vi "XLP80_EA_Close Devices.vi"(8 "err in":errorcluster, 10 "Device Informations":T1, 11 "Simu EAs":T2) -> (0 "Error EAs":T3)   [LabVIEW 2021]
uses:
  XLP80_EA_TDefsCluster_EA Setpoint.ctl
  XLP80_EA_TDefsCluster_EA Setpoint_Reku.ctl
  XLP80_EA_Globals.vi
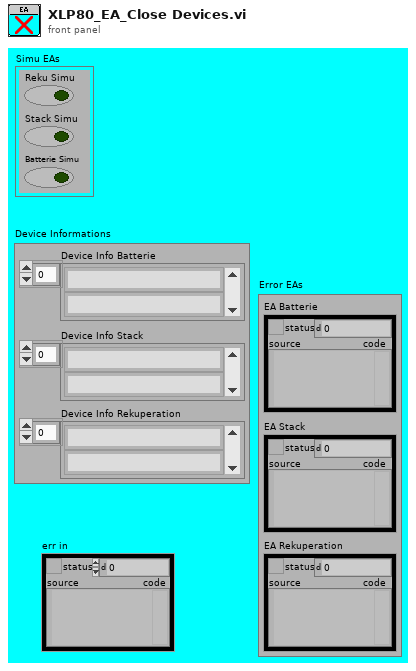
[diagram p1: front panel]
types:
  T1 = cluster{"Device Info Batterie":string[], "Device Info Stack":string[], "Device Info Rekuperation":string[]}
  T2 = cluster{"Reku Simu":bool, "Stack Simu":bool, "Batterie Simu":bool}
  T3 = cluster{"EA Batterie":errorcluster, "EA Stack":errorcluster, "EA Rekuperation":errorcluster}
  T4 = typedef "XLP80_EA_TDefsCluster_EA Setpoint_Reku.ctl" = cluster{"Load":bool, "Set Current":sgl, "Set Voltage":sgl, "Set Power":sgl}
  T5 = typedef "XLP80_EA_TDefsCluster_EA Setpoint.ctl" = cluster{"Load":bool, "Set Current":sgl, "Set Voltage":sgl}
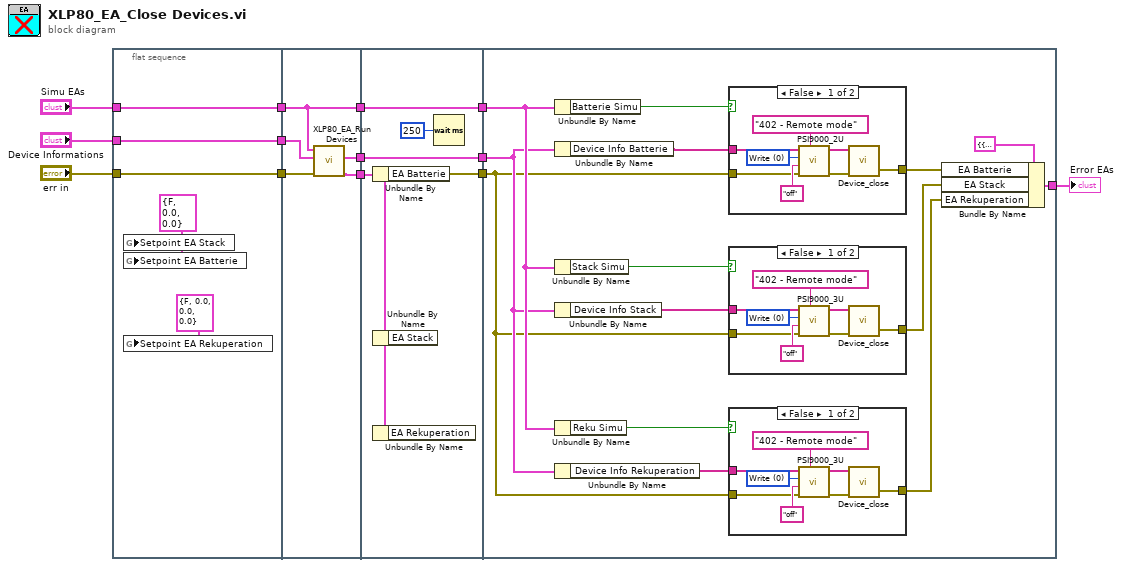
[diagram p0: block diagram]
diagram:
  n1 = flat-sequence {
    tunnel: "err in" -> [w16]
    tunnel: "Device Informations" -> [w17]
    tunnel: "Simu EAs" -> [w18]
    tunnel: [w18] -> w3
    tunnel: [w17] -> w2
    tunnel: [w16] -> w1
    tunnel: [w21] -> w6
    tunnel: [w20] -> w5
    tunnel: [w19] -> w4
    tunnel: w3 -> [w21]
    tunnel: w2 -> [w22]
    tunnel: w1 -> [w23]
    tunnel: [w28] -> w9
    tunnel: [w27] -> w8
    tunnel: [w26] -> w7
    tunnel: w6 -> [w28]
    tunnel: w5 -> [w27]
    tunnel: w4 -> [w25]
    tunnel: [w41] -> w13
    tunnel: w9 -> [w31]
    tunnel: w8 -> [w30]
    tunnel: w7 -> [w29]
    frame #0 {
      w15 = T5 {"Load"=FALSE, "Set Current"=0.0, "Set Voltage"=0.0} ("Setpoint EA Stack")
      n2 = global write "XLP80_EA_Globals.vi" "Setpoint EA Stack"(w15) -> ()
      n3 = global write "XLP80_EA_Globals.vi" "Setpoint EA Batterie"(w15) -> ()
      n4 = global write "XLP80_EA_Globals.vi" "Setpoint EA Rekuperation"(T4 {"Load"=FALSE, "Set Current"=0.0, "Set Voltage"=0.0, "Set Power"=0.0} ("Setpoint EA Rekuperation")) -> ()
    }
    frame #1 {
      n5 = call "XLP80_EA_Run Devices.vi"("err in"=w23, "Device Informations"=w22, "Simu EAs"=w21) -> ("Error EAs"=w19:T3, "Device Informations OUT"=w20:T1)  [unwired: 7 in]
    }
    frame #2 {
      n6 = Unbundle By Name(w25) -> ("EA Batterie"=w26:errorcluster)
      n7 = Unbundle By Name(w25) -> ()  [unwired: 1 out]
      n8 = Unbundle By Name(w25) -> ()  [unwired: 1 out]
      n9 = Wait (ms)(milliseconds to wait=u32 250) -> ()  [unwired: 1 out]
    }
    frame #3 {
      n10 = Unbundle By Name(w31) -> ("Batterie Simu"=w40:bool)
      n11 = Unbundle By Name(w30) -> ("Device Info Batterie"=w38:string[])
      n12 = Unbundle By Name(w31) -> ("Stack Simu"=w37:bool)
      n13 = Unbundle By Name(w30) -> ("Device Info Stack"=w36:string[])
      n14 = Unbundle By Name(w31) -> ("Reku Simu"=w33:bool)
      n15 = Unbundle By Name(w30) -> ("Device Info Rekuperation"=w34:string[])
      n16 = case shown="False" w40 {
        tunnel: [w68 w69] -> w39
        tunnel: w38 -> [w64 _]
        tunnel: w29 -> [w63 w69]
        frame False {
          w66 = u8 0 items=["Write", "Read"] ("Access")
          n17 = call <instrlib>:"PSI9000_2U.vi"("Command list"="402 - Remote mode", "Error in"=w63, "Value"="off", "Access"=w66, "Device information in"=w64) -> ("Error out"=w61:errorcluster, "Device information out"=w62:string[])  [unwired: 1 in, 2 out]
          n18 = call <instrlib>:"Device_close.vi"("error in (no error)"=w61, "Device information in"=w62) -> ("Fehler (Ausgang)"=w68:errorcluster)  [unwired: 3 in]
        }
        frame True {
        }
      }
      n19 = case shown="False" w37 {
        tunnel: [w59 w60] -> w35
        tunnel: w36 -> [w56 _]
        tunnel: w29 -> [w55 w60]
        frame False {
          w58 = u8 0 items=["Write", "Read"] ("Access")
          n20 = call <instrlib>:"PSI9000_3U.vi"("Command list"="402 - Remote mode", "Error in"=w55, "Value"="off", "Access"=w58, "Device information in"=w56) -> ("Error out"=w53:errorcluster, "Device information out"=w54:string[])  [unwired: 1 in, 2 out]
          n21 = call <instrlib>:"Device_close.vi"("error in (no error)"=w53, "Device information in"=w54) -> ("Fehler (Ausgang)"=w59:errorcluster)  [unwired: 3 in]
        }
        frame True {
        }
      }
      n22 = case shown="False" w33 {
        tunnel: [w50 w51] -> w32
        tunnel: w34 -> [w47 _]
        tunnel: w29 -> [w46 w51]
        frame False {
          w49 = u8 0 items=["Write", "Read"] ("Access")
          n23 = call <instrlib>:"PSI9000_3U.vi"("Command list"="402 - Remote mode", "Error in"=w46, "Value"="off", "Access"=w49, "Device information in"=w47) -> ("Error out"=w44:errorcluster, "Device information out"=w45:string[])  [unwired: 1 in, 2 out]
          n24 = call <instrlib>:"Device_close.vi"("error in (no error)"=w44, "Device information in"=w45) -> ("Fehler (Ausgang)"=w50:errorcluster)  [unwired: 3 in]
        }
        frame True {
        }
      }
      n25 = Bundle By Name(cluster=T3 {"EA Batterie"={"status"=FALSE, "code"=0, "source"=""}, "EA Stack"={"status"=FALSE, "code"=0, "source"=""}, "EA Rekuperation"={"status"=FALSE, "code"=0, "source"=""}} ("Error EAs"), "EA Batterie"=w39, "EA Stack"=w35, "EA Rekuperation"=w32) -> (w41:T3)
    }
  }
  "Error EAs" <- w13
